vi "testNotificationDll.vi"() -> ()   [LabVIEW 2011]
panel:
  out "通知":string
  in  "s":string
  in  "布尔":bool
  out "数值 2":i32
  out "数值":i32
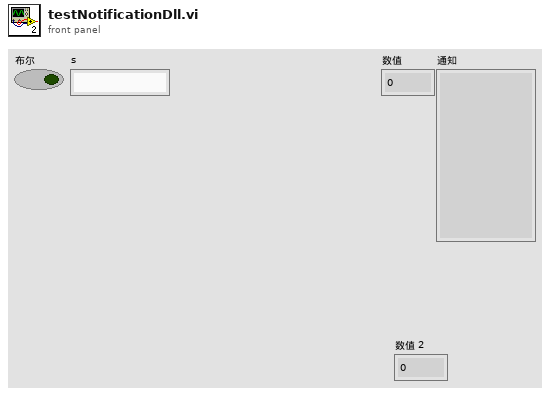
[diagram p1: front panel]
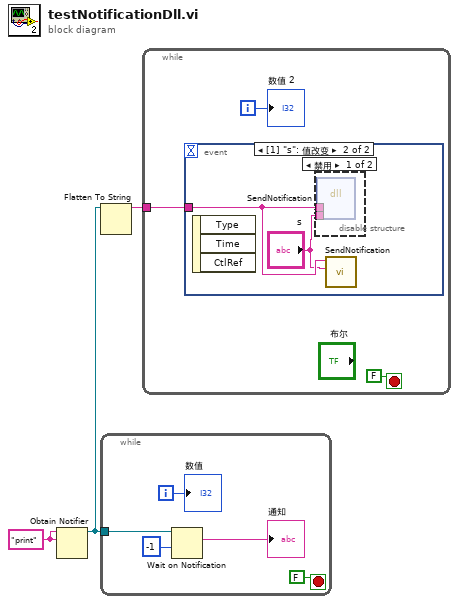
[diagram p0: block diagram]
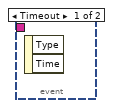
[diagram p2: hidden frame]
diagram:
  w3 = "print" ("name")
  n1 = Obtain Notifier(name (unnamed)=w3, notification data type=w3) -> (notifier out=w1:refnum<notifier>)  [unwired: 2 in, 2 out]
  n2 = Flatten To String(anything=w1) -> (data string=w2:string)  [unwired: 3 in, 2 out]
  n3 = while {
    tunnel: w1 -> [w4]
    i -> [w7]
    stop <- FALSE stop-if-true
    n4 = Wait on Notification(notifier=w4, timeout in ms (-1)=-1 ("timeup")) -> (notification=→"通知":string)  [unwired: 2 in, 3 out]
    "数值" <- w7
  }
  n5 = while {
    tunnel: w2 -> [w9]
    i -> [w10]
    stop <- FALSE stop-if-true
    n6 = event shown="[1] \"s\": 值改变" {
      selector: _ -> [_ _]
      dyn-events: _ -> [_ _]
      timeout: _ -> [_ _]
      tunnel: w9 -> [_ w13]
      event Timeout {
        n7 = event-data() -> ()  [unwired: 1 in, 2 out]
      }
      event "s": Value Change {
        n8 = event-data() -> ()  [unwired: 1 in, 3 out]
        n9 = disable-structure shown="禁用" {
          disable-tunnel: w13 -> [w15 _]
          disable-tunnel: "s" -> [w14 _]
          frame Disabled {
            n10 = dll-call lib="PTH1Nabs GworkLuaDllToLabviewbuilds\ttestC_dll\t我的DLLNotification.dll" fn="SendNotification"("s"=w15, "Notification"=w14) -> ()  [unwired: 6 in, 2 out]
          }
          frame Enabled {
          }
        }
        n11 = call "SendNotification.vi"("notification"=w13, "s"="s") -> ()  [unwired: 9 in]
      }
    }
    "数值 2" <- w10
  }
